vi "RPS_MAIN para ver en tiempo real cambios en la curva.vi"() -> ()   [LabVIEW 2013]
panel:
  in  "Espesores (angstroms)":dbl[](array[slide]) scale=0.0..1000.0
  in  "Número de capas":u32=1
  in  "q máximo":dbl=90.0
  in  "q mínimo":dbl=30.0
  in  "Resolución":dbl=1000.0
  in  "l(angstroms)":dbl=6328.0
  in  "Coeficientes de extinción":dbl[](array[slide]) scale=-5.0..5.0
  in  "Índices de refracción":dbl[](array[slide]) scale=0.0..10.0
  out "q RPS":dbl
  in  "SALIR DEL PROGRAMA":bool
  out "Curva RPS":cluster{"q0r":dbl[], dbl[]}(graph)
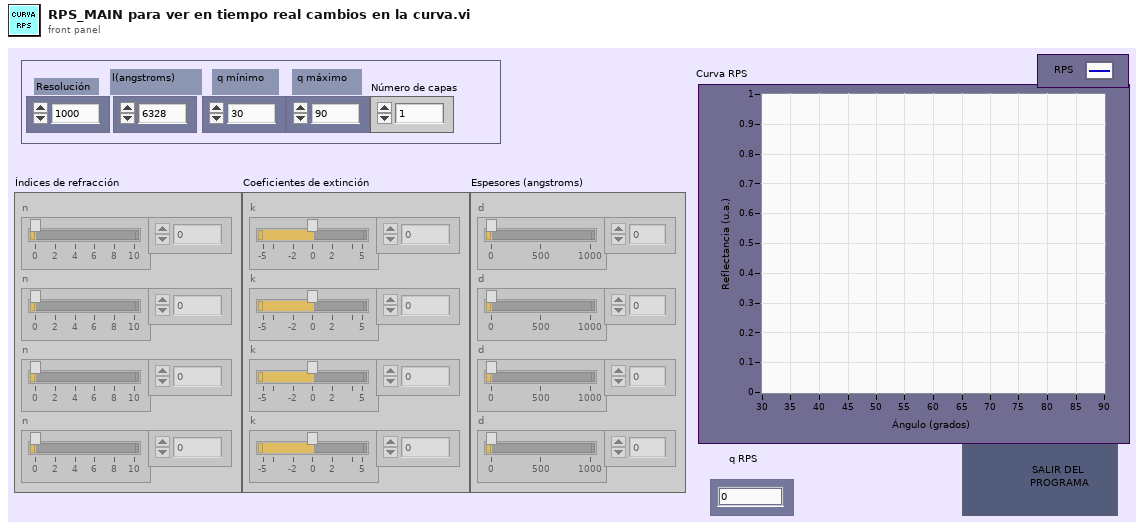
[diagram p1: front panel]
types:
  T1 = typedef "NI_Matrix.lvlib/ComplexMatrix.ctl" = cdb[][]
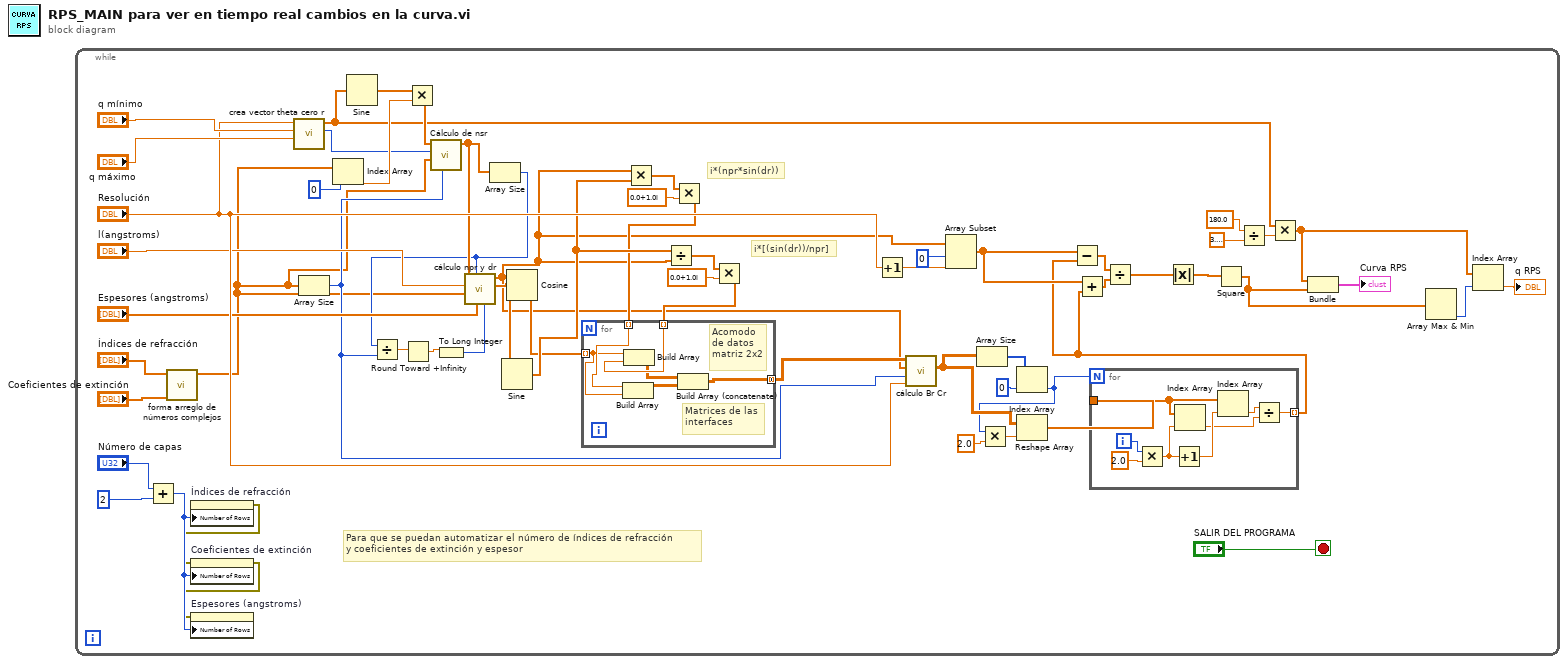
[diagram p0: block diagram]
diagram:
  n1 = while {
    stop <- "SALIR DEL PROGRAMA" stop-if-true
    # "i*[(sin(dr))/npr]"
    # "i*(npr*sin(dr))"
    # "Para que se puedan automatizar el número de índices de refracción\ny coeficientes de extinción y espesor"
    n2 = Add(x="Número de capas", y=u32 2) -> (x+y=w6:u32)
    n3 = call "forma arreglo de números complejos.vi"("Coeficientes de extinción"="Coeficientes de extinción", "Índices de refracción"="Índices de refracción") -> ("n + ik"=w7:cdb[])  [unwired: 9 in]
    n4 = property on="Índices de refracción" class="Arr (strict)"("Number of Rows"=w6) -> (error out=w3:errorcluster)  [unwired: 2 in, 1 out]
    n5 = property on="Coeficientes de extinción" class="Arr (strict)"(error in=w3, "Number of Rows"=w6) -> (error out=w2:errorcluster)  [unwired: 1 in, 1 out]
    n6 = property on="Espesores (angstroms)" class="Arr (strict)"(error in=w2, "Number of Rows"=w6) -> ()  [unwired: 1 in, 2 out]
    n7 = call "crea vector theta cero r.vi"("q máximo"="q máximo", "q mínimo"="q mínimo", "Resolución"="Resolución") -> ("Tamaño (r)"=w45:i32, "q0r"=w10:dbl[])  [unwired: 6 in, 1 out]
    n8 = Array Size(array=w7) -> (size(s)=w29:i32)
    n9 = Index Array(array=w7, index=0) -> (element=w46:cdb)
    n10 = Sine(x=w10) -> (sin(x)=w47:dbl[])
    n11 = Multiply(x=w47, y=w46) -> (x*y=w44:cdb[])
    n12 = call "Cálculo de nsr.vi"(">>tn>>"=w29, ">>n[]>>"=w7, "Tamaño (r)"=w45, ">>sr>>"=w44) -> (">>nsr>>"=w43:cdb[])  [unwired: 7 in]
    n13 = Array Size(array=w43) -> (size(s)=w31:i32)
    n14 = Divide(x=w31, y=w29) -> (x/y=w42:dbl)
    n15 = Round Toward +Infinity(x=w42) -> (ceil(x): smallest int >= x=w41:dbl)
    n16 = To Long Integer(number=w41) -> (32bit integer=w9:i32)
    n17 = call "cálculo npr y dr.vi"("Numeric Control"=w9, ">>d>>"="Espesores (angstroms)", "Numeric Control 2"=w31, ">>n[]>>"=w7, ">>lambda>>"="l(angstroms)", ">>nsr>>"=w43) -> (">>dr>>"=w40:cdb[], ">>nPr>>"=w21:csg[])  [unwired: 4 in]
    n18 = Sine(x=w40) -> (sin(x)=w37:cdb[])
    n19 = Cosine(x=w40) -> (cos(x)=w34:cdb[])
    n20 = Multiply(x=w21, y=w37) -> (x*y=w39:cdb[])
    n21 = Divide(x=w37, y=w21) -> (x/y=w36:cdb[])
    n22 = Multiply(x=w39, y=csg 0.0+1.0i) -> (x*y=w32:cdb[])
    n23 = Multiply(x=w36, y=csg 0.0+1.0i) -> (x*y=w33:cdb[])
    n24 = for {
      tunnel: [w74] -> w30 mode=concatenating
      tunnel: w34 -> [w71] mode=indexing
      tunnel: w33 -> [w73] mode=indexing
      tunnel: w32 -> [w72] mode=indexing
      # "Matrices de las\ninterfaces"
      # "Acomodo\nde datos\nmatriz 2x2"
      n25 = Build Array(w72, w71) -> (w69:T1)
      n26 = Build Array(w71, w73) -> (w70:T1)
      n27 = Build Array (concatenate)(w70, w69) -> (w74:T1)
    }
    n28 = Increment(x="Resolución") -> (x+1=w19:dbl)
    n29 = call "cálculo Br Cr.vi"("Resolución"="Resolución", "Número de índices de refracción"=w29, "npr"=w21, "Matrices interfaces"=w30) -> ("Br\nCr"=w28:cdb[][][])  [unwired: 4 in, 3 out]
    n30 = Array Subset(array=w21, index=0, length=w19) -> (w18:csg[])
    n31 = Array Size(array=w28) -> (size(s)=w27:i32[])
    n32 = Index Array(array=w27, index=0) -> (element=w22:i32)
    n33 = Multiply(x=w22, y=2.0) -> (x*y=w23:dbl)
    n34 = Reshape Array(w28, w23) -> (w24:cdb[])
    n35 = for {
      N: w22 -> [_]
      tunnel: w24 -> [w66]
      tunnel: [w61] -> w5 mode=indexing
      i -> [w67]
      n36 = Multiply(x=w67, y=2.0) -> (x*y=w65:dbl)
      n37 = Increment(x=w65) -> (x+1=w64:dbl)
      n38 = Index Array(array=w66, index=w65) -> (element=w62:cdb)
      n39 = Index Array(array=w66, index=w64) -> (element=w63:cdb)
      n40 = Divide(x=w63, y=w62) -> (x/y=w61:cdb)
    }
    n41 = Subtract(x=w18, y=w5) -> (x-y=w17:cdb[])
    n42 = Add(x=w18, y=w5) -> (x+y=w16:cdb[])
    n43 = Divide(x=w17, y=w16) -> (x/y=w15:cdb[])
    n44 = Absolute Value(x=w15) -> (abs(x)=w14:dbl[])
    n45 = Square(x=w14) -> (x^2=w49:dbl[])
    n46 = Divide(x=180.0, y=3.141592653589793) -> (x/y=w11:dbl)
    n47 = Multiply(x=w10, y=w11) -> (x*y=w50:dbl[])
    n48 = Bundle(w50, w49) -> (→"Curva RPS":cluster{dbl[], dbl[]})  [unwired: 1 in]
    n49 = Array Max & Min(array=w49) -> (min index (indices)=w8:i32)  [unwired: 3 out]
    n50 = Index Array(array=w50, index=w8) -> (element=→"q RPS":dbl)
  }
